vi "IsConnected.vi"(8 "error in (no error)":errorcluster, 11 "MultiReader in":refnum<class "MultiReader.lvclass">) -> (0 "error out":errorcluster, 2 "connected?":bool, 3 "MultiReader out":refnum<class "MultiReader.lvclass">)   [LabVIEW 2025, in "MultiReader.lvclass"]
doc: "Returns TRUE if the Readers connection is alive"
uses:
  MultiReader.lvclass
  MultiReader.lvclass/MultiReader.ctl
  BaseReader/BaseReader.lvclass
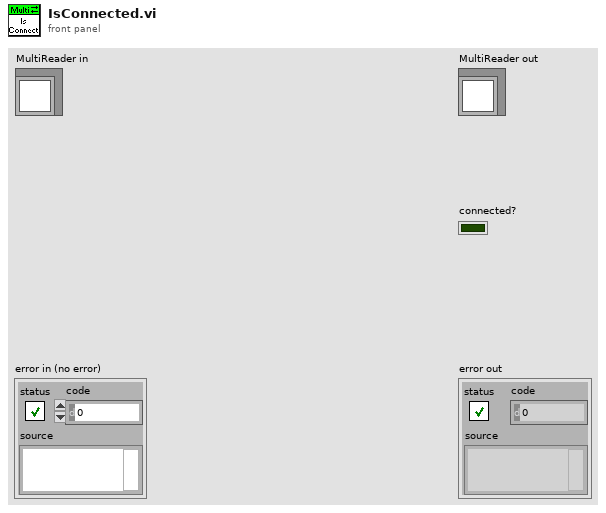
[diagram p1: front panel]
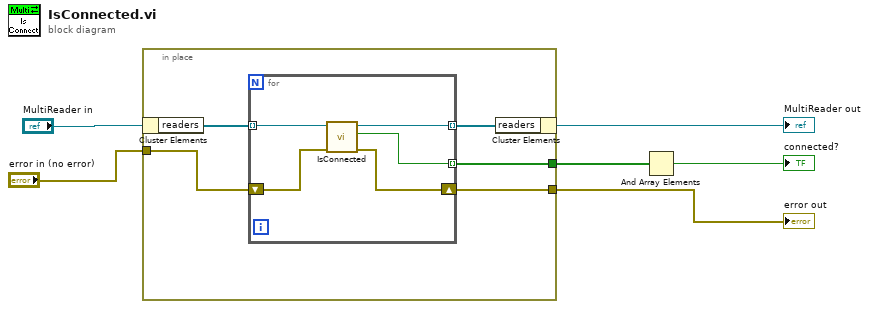
[diagram p0: block diagram]
diagram:
  n1 = in-place {
    in-place-border: [w9] -> w4
    in-place-border: "error in (no error)" -> [w8]
    in-place-border: [w7] -> w2
    n2 = in-place-cluster #1("MultiReader in") -> ("readers"=w11:refnum<class "BaseReader.lvclass">[])
    n3 = for {
      tunnel: w11 -> [w16] mode=indexing
      tunnel: [w15] -> w10 mode=indexing
      shift-right: [w13] -> w9
      shift-left: w8 -> [w14]
      tunnel: [w12] -> w7 mode=indexing
      n4 = call-dynamic "IsConnected.vi"("error in (no error)"=w14, "BaseReader in"=w16) -> ("error out"=w13:errorcluster, "connected?"=w12:bool, "BaseReader out"=w15:refnum<class "BaseReader.lvclass">)  [unwired: 7 in]
    }
    n5 = in-place-cluster #1("readers"=w10) -> (→"MultiReader out":refnum<class "MultiReader.lvclass">)
  }
  "error out" <- w4
  n6 = And Array Elements(Boolean array=w2) -> (logical AND=→"connected?":bool)
